vi "fmt_writeFormatBufferHeaders.vi"(8 "error in (no error)":errorcluster, 11 "Format buffers in":T1) -> (0 "error out":errorcluster, 3 "Format buffers out":T1)   [LabVIEW 2020, in "NI_ExcelFile.lvlib"]
uses:
  <vilib>/express/express shared/NI_ExcelFile/NI_ExcelFile.lvlib
  <vilib>/express/express shared/NI_ExcelFile/Ctrls/fmt_formatBuffer.ctl
  <vilib>/express/express shared/NI_ExcelFile/Ctrls/TimeColumnMode.ctl
  <vilib>/express/express shared/NI_ExcelFile/Ctrls/Columns.ctl
  <vilib>/express/express shared/NI_ExcelFile/Ctrls/ColumnInfo.ctl
  <vilib>/express/express shared/NI_ExcelFile/Ctrls/DataType.ctl
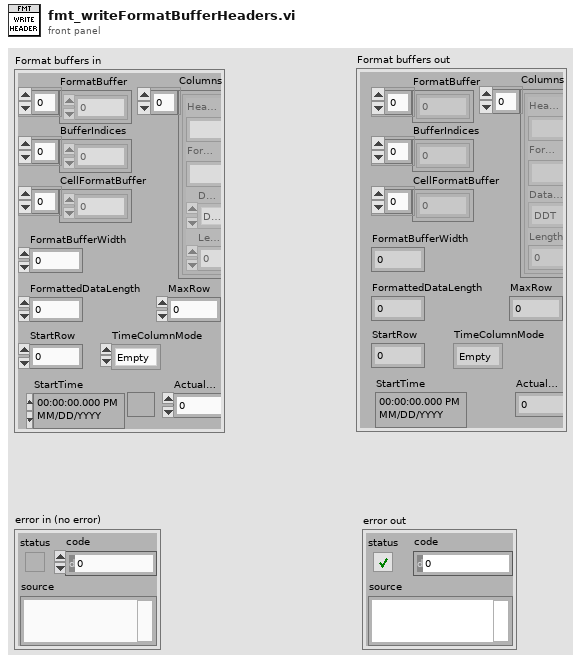
[diagram p1: front panel]
types:
  T1 = typedef "NI_ExcelFile.lvlib/fmt_formatBuffer.ctl" = cluster{"FormatBuffer":u8[], "BufferIndices":i32[], "CellFormatBuffer":u8[], "FormatBufferWidth":i32, "FormattedDataLength":i32, "MaxRow":i32, "StartRow":i32, "TimeColumnMode":T2, "StartTime":timestamp, "Columns":T3, "ActualLength":i32}
  T2 = typedef "NI_ExcelFile.lvlib/TimeColumnMode.ctl" = enum16{"Empty", "OnePerCh", "One"}
  T3 = typedef "NI_ExcelFile.lvlib/Columns.ctl" = T4[]
  T4 = typedef "NI_ExcelFile.lvlib/ColumnInfo.ctl" = cluster{"Header":string, "Format":string, "DataType":T5, "Length":u64}
  T5 = typedef "NI_ExcelFile.lvlib/DataType.ctl" = enum16{"DDT", "WFM", "Array of STR", "Array of DBL", "Array of I8", "Array of I16", "Array of I32", "Array of I64", "Array of SGL", "Array of U8", "Array of U16", "Array of U32", "Array of U64", "Array of Time"}
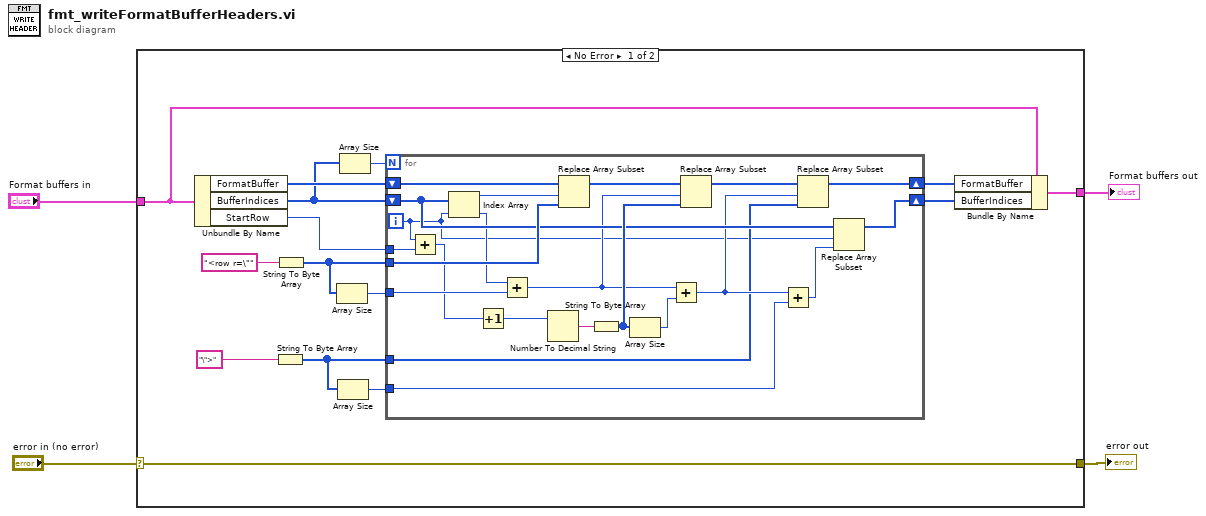
[diagram p0: block diagram]
diagram:
  n1 = case shown="No Error" "error in (no error)" {
    selector: "error in (no error)" -> [w5 w41]
    tunnel: [w18 w42] -> w4
    tunnel: "Format buffers in" -> [w17 w42]
    tunnel: [w5 w41] -> w1
    frame No Error {
      n2 = Unbundle By Name(w17) -> ("FormatBuffer"=w19:u8[], "BufferIndices"=w10:i32[], "StartRow"=w6:i32)
      n3 = String To Byte Array(string="\">") -> (unsigned byte array=w8:u8[])
      n4 = String To Byte Array(string="<row r=\"") -> (unsigned byte array=w13:u8[])
      n5 = Array Size(array=w13) -> (size(s)=w12:i32)
      n6 = Array Size(array=w8) -> (size(s)=w7:i32)
      n7 = Array Size(array=w10) -> (size(s)=w11:i32)
      n8 = for {
        N: w11 -> [_]
        shift-right: [w26] -> w16
        shift-left: w19 -> [w40]
        shift-right: [w34] -> w15
        shift-left: w10 -> [w33]
        tunnel: w13 -> [w39]
        tunnel: w12 -> [w38]
        tunnel: w8 -> [w24]
        tunnel: w7 -> [w28]
        tunnel: w6 -> [w21]
        i -> [w20]
        n9 = Add(x=w20, y=w21) -> (x+y=w22:i32)
        n10 = Index Array(array=w33, index=w20) -> (element=w23:i32)
        n11 = Increment(x=w22) -> (x+1=w30:i32)
        n12 = Add(x=w23, y=w38) -> (x+y=w32:i32)
        n13 = Number To Decimal String(number=w30) -> (decimal integer string=w37:string)  [unwired: 1 in]
        n14 = Replace Array Subset(array=w40, new element=w39, index=w23) -> (w36:u8[])
        n15 = String To Byte Array(string=w37) -> (unsigned byte array=w35:u8[])
        n16 = Array Size(array=w35) -> (size(s)=w31:i32)
        n17 = Add(x=w32, y=w31) -> (x+y=w25:i32)
        n18 = Replace Array Subset(array=w36, new element=w35, index=w32) -> (w27:u8[])
        n19 = Add(x=w25, y=w28) -> (x+y=w29:i32)
        n20 = Replace Array Subset(array=w27, new element=w24, index=w25) -> (w26:u8[])
        n21 = Replace Array Subset(array=w33, new element=w29, index=w20) -> (w34:i32[])
      }
      n22 = Bundle By Name(cluster=w17, "FormatBuffer"=w16, "BufferIndices"=w15) -> (w18:T1)
    }
    frame Error {
    }
  }
  "Format buffers out" <- w4
  "error out" <- w1
